vi "UDPStateReceiver.vi"() -> ()   [LabVIEW 2018]
uses:
  Library/Simple UDP Message/Simple UDP Message.lvlib
panel:
  out "data out":string
  out "iteration":i32
  in  "Stop":bool
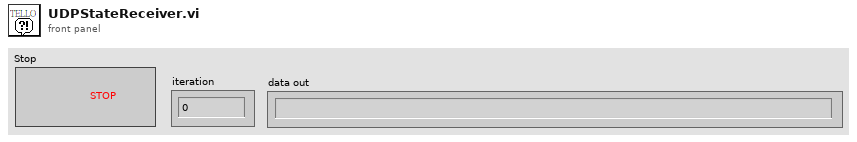
[diagram p1: front panel]
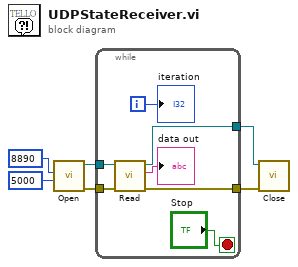
[diagram p0: block diagram]
diagram:
  n1 = call "Open.vi"("timeout ms (60000)"=5000 ("timeout ms (25000)"), "port"=u16 8890) -> ("error out"=w2:errorcluster, "connection ID"=w1:refnum<k16>)  [unwired: 8 in]
  n2 = while {
    tunnel: w2 -> [w10]
    tunnel: [w9] -> w4
    tunnel: [w8] -> w3
    tunnel: w1 -> [w7]
    i -> [w12]
    stop <- "Stop" stop-if-true
    n3 = call "Read.vi"("error in (no error)"=w10, "connection ID"=w7) -> ("error out"=w9:errorcluster, "data out"=→"data out":string, "connection ID"=w8:refnum<k16>)  [unwired: 5 in, 2 out]
    "iteration" <- w12
  }
  n4 = call "Close.vi"("error in (no error)"=w4, "connection ID"=w3) -> ()  [unwired: 9 in, 1 out]
